vi "start_sweep.vi"(8 "error in (no error)":errorcluster, 11 "ScanModeTS090821Circular2D in":refnum<class "ImagingModeTS090821Circular2D.lvclass">) -> (0 "error out":errorcluster, 3 "ScanModeTS090821Circular2D out":refnum<class "ImagingModeTS090821Circular2D.lvclass">)   [LabVIEW 2010, in "ImagingModeTS090821Circular2D.lvclass"]
uses:
  ImagingModeTS090821Circular2D.lvclass
  ImagingModeTS090821Circular2D.lvclass/ImagingModeTS090821Circular2D.ctl
  ImagingModeDL091001Scaffold/ImagingModeDL091001Scaffold/ImagingModeDL091001Scaffold.lvclass
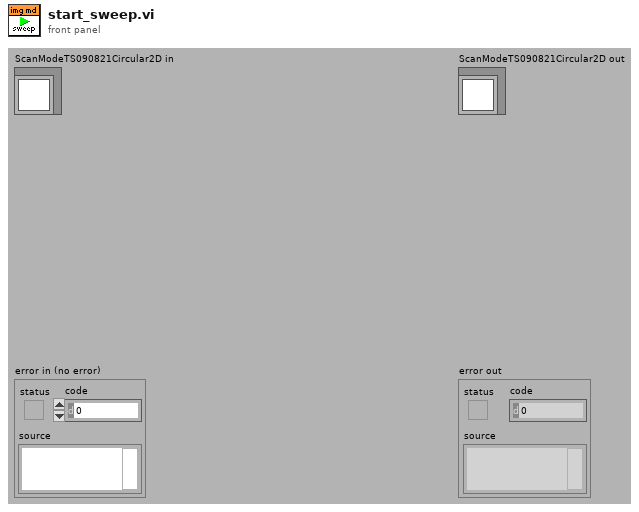
[diagram p1: front panel]
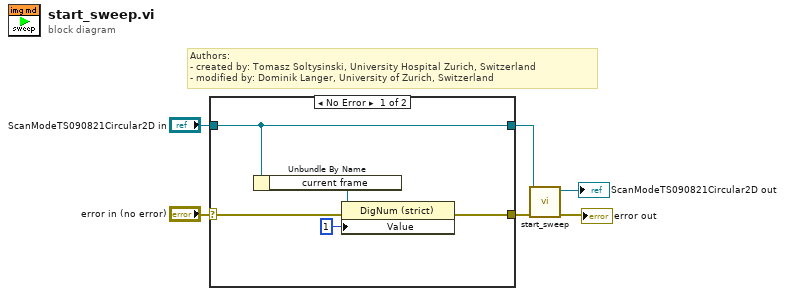
[diagram p0: block diagram]
diagram:
  # "Authors: \n- created by: Tomasz Soltysinski, University Hospital Zurich, Switzerland\n- modified by: Dominik Langer, University of Zurich, Switzerland"
  n1 = case shown="No Error" "error in (no error)" {
    selector: "error in (no error)" -> [w9 w13]
    tunnel: [w8 w13] -> w3
    tunnel: [w11 w12] -> w1
    tunnel: "ScanModeTS090821Circular2D in" -> [w11 w12]
    frame No Error {
      n2 = Unbundle By Name(w11) -> ("current frame"=w10:refnum<vi>)
      n3 = property class="DigNum (strict)"(reference=w10, error in=w9, "Value"=1) -> (error out=w8:errorcluster)  [unwired: 1 out]
    }
    frame Error {
    }
  }
  n4 = call-parent "start_sweep.vi"("error in (no error)"=w3, "ScanModeDL091001Scaffold in"=w1) -> ("error out"=→"error out":errorcluster, "ScanModeDL091001Scaffold out"=→"ScanModeTS090821Circular2D out":refnum<class "ImagingModeTS090821Circular2D.lvclass">)  [unwired: 8 in]
